vi "Create.vi"(8 "error in (no error)":errorcluster, 10 "Result":refnum<class "Result.lvclass">) -> (0 "error out":errorcluster, 3 "Promise out":refnum<class "Promise.lvclass">)   [LabVIEW 2017, in "Futures.lvlib" / "Promise.lvclass"]
uses:
  Promise.lvclass
  Result/Result.lvclass
  Promise.lvclass/Promise.ctl
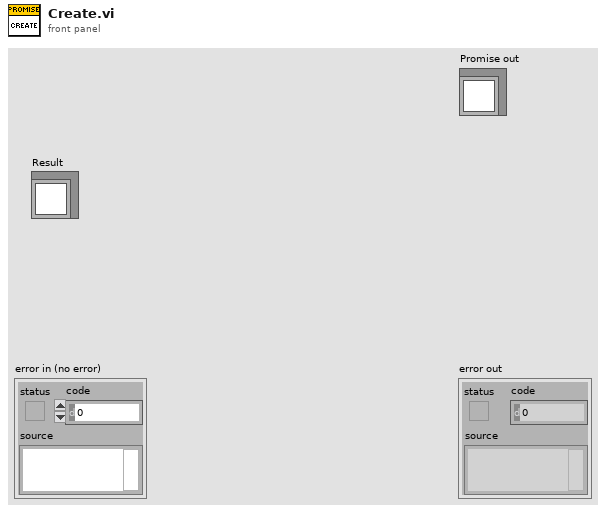
[diagram p1: front panel]
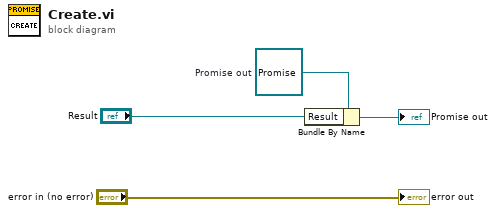
[diagram p0: block diagram]
diagram:
  w4 = refnum<class "Promise.lvclass"> refnum  # Promise out
  n1 = Bundle By Name(cluster=w4, "Result"="Result") -> (→"Promise out":refnum<class "Promise.lvclass">)
  "error out" <- "error in (no error)"
